vi "PPMS.setTemperature.vi"(8 "error in (no error)":errorcluster, 10 "Data":variant, 11 "instrument.PPMS":refnum<class "instrument.PPMS.lvclass">) -> (0 "error out":errorcluster, 3 "instrument.PPMS out":refnum<class "instrument.PPMS.lvclass">)   [LabVIEW 2019, in "instrument.PPMS.lvclass"]
uses:
  instrument.PPMS.lvclass
  <userlib>/LevyLab/Instrument Framework/Instrument Types/Cryostat/Typedefs/setTemperature--cluster.ctl
  instrument.PPMS.lvclass/instrument.PPMS.ctl
  4008bc7a-1f3a-4de3-b431-581da613ca51.vi
  4008bc7a-1f3a-4de3-b431-581da613ca51.vi/c9e9bb1d-9846-411c-bb71-14d429dfadcd.vi
  4008bc7a-1f3a-4de3-b431-581da613ca51.vi/4f8b7b58-adf5-4077-bbdd-5efcc1aefa91.vi
  <vilib>/Utility/Data Type/Get Type Information.vi
  <vilib>/JDP Science/JSONtext/JSON text to Variant.vi
  <vilib>/JDP Science/JSONtext/LVClass Serializer/JSONtext LVClass Serializer.lvclass
  <userlib>/LevyLab/Instrument Framework/Instrument Types/Cryostat/Instrument.Cryostat.lvclass
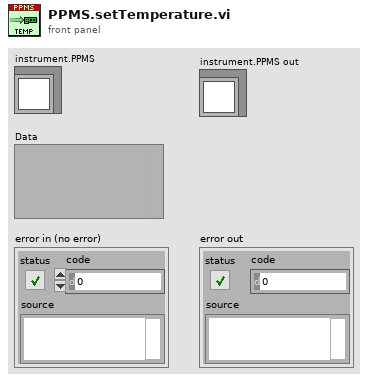
[diagram p1: front panel]
types:
  T1 = typedef "Instrument.Cryostat.lvclass/setTemperature--cluster.ctl" = cluster{"temperature":dbl, "rate":dbl, "channel":i32}
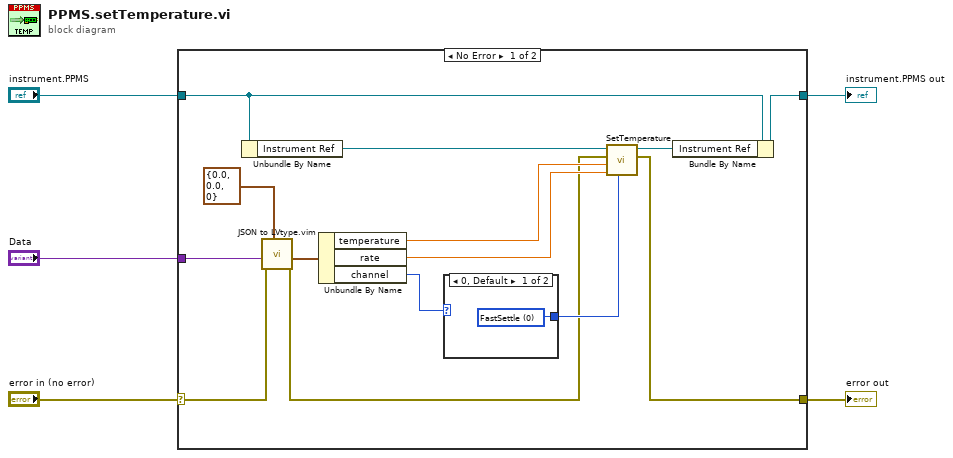
[diagram p0: block diagram]
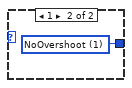
[diagram p2: hidden frame]
diagram:
  n1 = case shown="No Error" "error in (no error)" {
    selector: "error in (no error)" -> [w7 w23]
    tunnel: "Data" -> [w8 _]
    tunnel: [w18 w23] -> w4
    tunnel: "instrument.PPMS" -> [w12 w22]
    tunnel: [w13 w22] -> w2
    frame No Error {
      n2 = Unbundle By Name(w12) -> ("Instrument Ref"=w17:refnum<k24>)
      n3 = call "JSON to LVtype.vim"("type"=T1 {"temperature"=0.0, "rate"=0.0, "channel"=0} ("Set Temperature"), "error in (no error)"=w7, "JSON Data in"=w8) -> ("error out"=w9:errorcluster, "Data out"=w10:T1)  [unwired: 7 in]
      n4 = Unbundle By Name(w10) -> ("temperature"=w15:dbl, "rate"=w14:dbl, "channel"=w6:i32)
      n5 = case shown="0, Default" w6 {
        tunnel: [w20 w21] -> w19
        frame 0, Default {
          w20 = 0 items=["FastSettle", "NoOvershoot"] ("Approach")
        }
        frame 1 {
          w21 = 1 items=["FastSettle", "NoOvershoot"] ("Approach")
        }
      }
      n6 = call "SetTemperature.vi"("Approach"=w19, "Rate"=w14, "Temperature"=w15, "error in (no error)"=w9, "Instrument Ref In"=w17) -> ("error out"=w18:errorcluster, "Instrument Ref Out"=w11:refnum<k24>)  [unwired: 2 in, 1 out]
      n7 = Bundle By Name(cluster=w12, "Instrument Ref"=w11) -> (w13:refnum<class "instrument.PPMS.lvclass">)
    }
    frame Error {
    }
  }
  "error out" <- w4
  "instrument.PPMS out" <- w2
